vi "q3w5.vi"() -> ()   [LabVIEW 2015]
uses:
  <vilib>/LabVIEW Interface for Arduino/LabVIEW Interface for Arduino.lvlib
panel:
  out "Numeric":dbl format="%#_13g"
  in  "stop":bool
  in  "VISA resource":refnum<visa-resource-name>
  in  "Your Answer":dbl
  in  "Second":i32
  in  "First":i32
  in  "Enum":enum16{"Divide", "Multiply", "Subtract", "Add"}(ring)
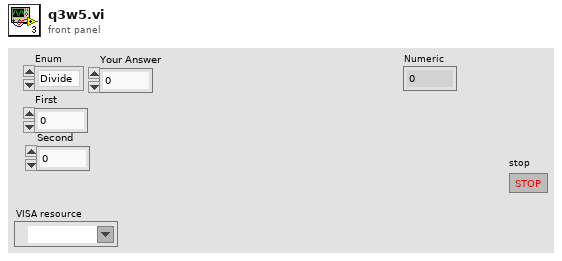
[diagram p1: front panel]
types:
  T1 = typedef "LabVIEW Interface for Arduino.lvlib/Arduino Resource.ctl" = cluster{"VISA resource":refnum<visa-resource-name>, "Board Type":T2, "Connection Type":enum8{"USB / Serial"}, "Bytes Per Packet (15)":u8}
  T2 = typedef "LabVIEW Interface for Arduino.lvlib/Board Type.ctl" = enum16{"Uno", "Dimuelanove w/Atmega 328", "Mega 2560"}
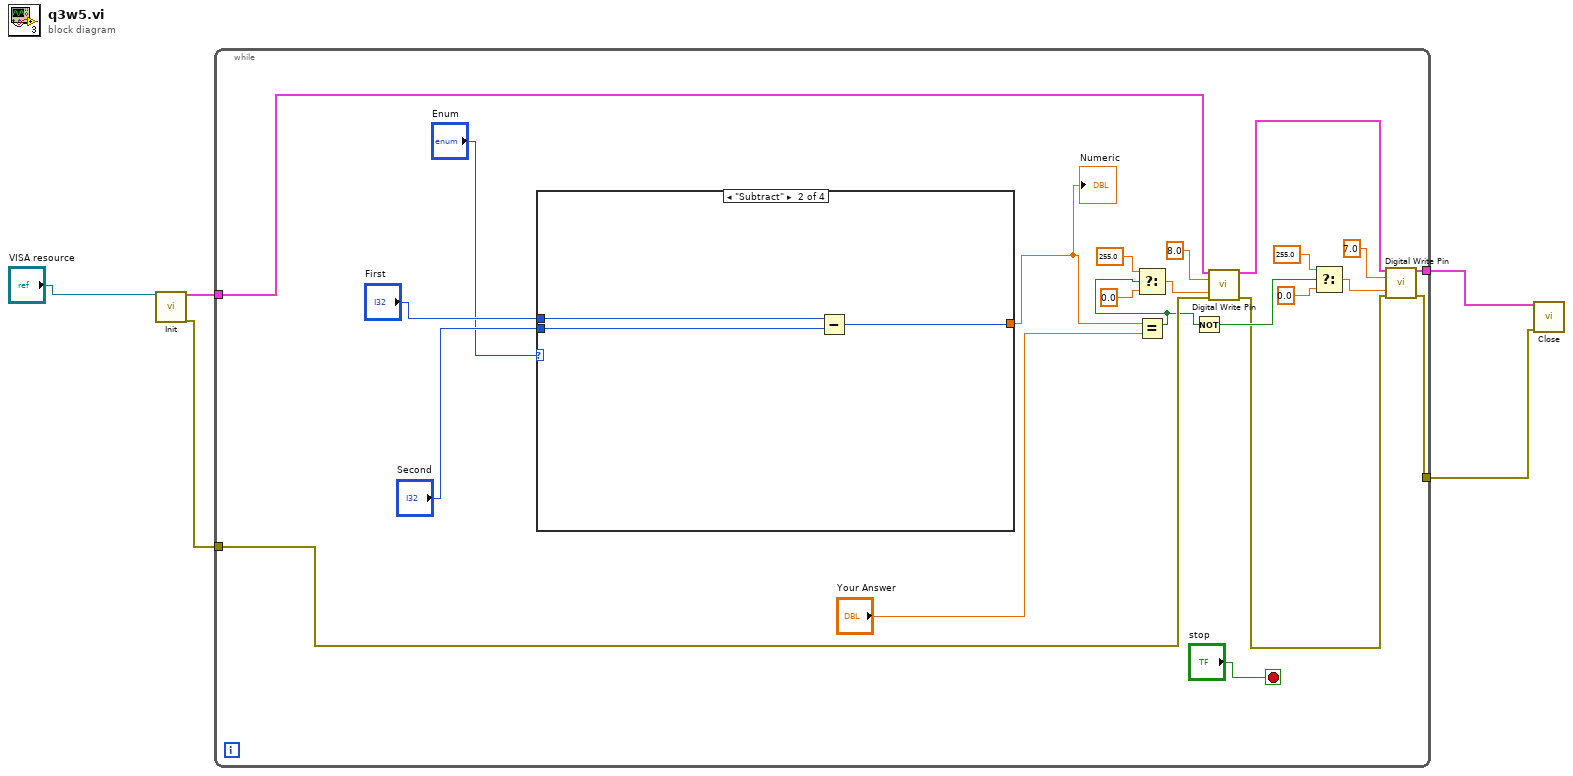
[diagram p0: block diagram]
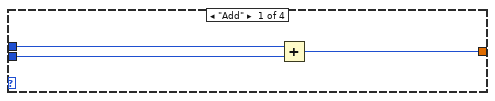
[diagram p2: hidden frame]
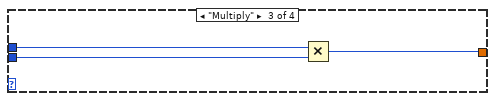
[diagram p3: hidden frame]
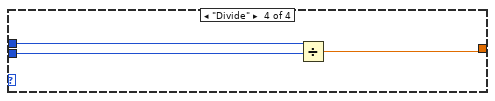
[diagram p4: hidden frame]
diagram:
  n1 = call <vilib>:"Init.vi"("VISA resource"="VISA resource") -> ("Arduino Resource"=w4:T1, "error out"=w3:errorcluster)  [unwired: 17 in]
  n2 = while {
    tunnel: w4 -> [w21]
    tunnel: w3 -> [w22]
    tunnel: [w7] -> w2
    tunnel: [w6] -> w1
    stop <- "stop" stop-if-true
    n3 = case shown="\"Subtract\"" "Enum" {
      tunnel: "First" -> [w30 w33 w36 w39]
      tunnel: "Second" -> [w29 w32 w35 w37]
      tunnel: [w28 w31 w34 w38] -> w16
      frame "Add" {
        n4 = Add(x=w30, y=w29) -> (x+y=w28:i32)
      }
      frame "Subtract" {
        n5 = Subtract(x=w33, y=w32) -> (x-y=w31:i32)
      }
      frame "Multiply" {
        n6 = Multiply(x=w36, y=w35) -> (x*y=w34:i32)
      }
      frame "Divide" {
        n7 = Divide(x=w39, y=w37) -> (x/y=w38:dbl)
      }
    }
    "Numeric" <- w16
    n8 = Equal?(x=w16, y="Your Answer") -> (x = y?=w15:bool)
    n9 = Select(t=255.0, s=w15, f=0.0) -> (s? t:f=w24:dbl)
    n10 = Not(x=w15) -> (.not. x?=w10:bool)
    n11 = call <vilib>:"Digital Write Pin.vi"("Arduino Resource"=w21, "Digital I/O Pin (0)"=8.0, "Value (0)"=w24, "error in"=w22) -> ("Arduino Resource"=w9:T1, "error out"=w8:errorcluster)  [unwired: 10 in]
    n12 = Select(t=255.0, s=w10, f=0.0) -> (s? t:f=w12:dbl)
    n13 = call <vilib>:"Digital Write Pin.vi"("Arduino Resource"=w9, "Digital I/O Pin (0)"=7.0, "Value (0)"=w12, "error in"=w8) -> ("Arduino Resource"=w6:T1, "error out"=w7:errorcluster)  [unwired: 10 in]
  }
  n14 = call <vilib>:"Close.vi"("Arduino Resource"=w1, "error in"=w2) -> ()  [unwired: 13 in, 1 out]
